vi "Get Target Info.vi"(8 "error in (no error)":errorcluster, 11 "FileOperation in":refnum<class "FileOperation.lvclass">) -> (0 "error out":errorcluster, 3 "FileOperation out":refnum<class "FileOperation.lvclass">)   [LabVIEW 2015, in "FileOperation.lvclass"]
uses:
  FileOperation.lvclass
  FileOperation.lvclass/FileOperation.ctl
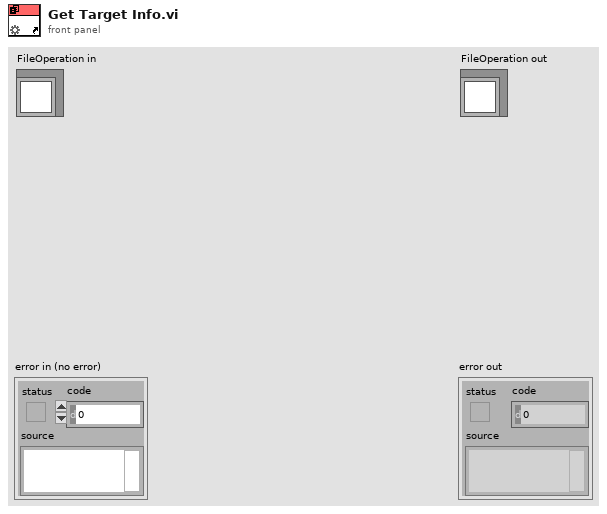
[diagram p1: front panel]
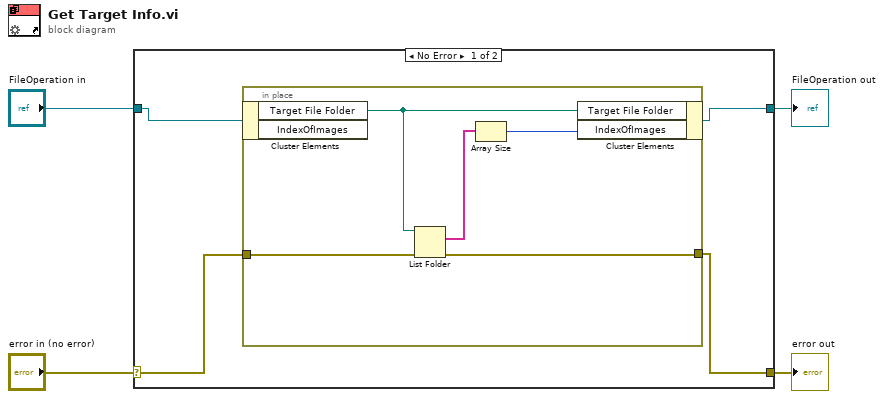
[diagram p0: block diagram]
diagram:
  n1 = case shown="No Error" "error in (no error)" {
    selector: "error in (no error)" -> [w8 w15]
    tunnel: [w6 w15] -> w3
    tunnel: [w5 w14] -> w1
    tunnel: "FileOperation in" -> [w7 w14]
    frame No Error {
      n2 = in-place {
        in-place-border: w8 -> [w13]
        in-place-border: [w10] -> w6
        n3 = in-place-cluster #1(w7) -> ("Target File Folder"=w12:path)  [unwired: 1 out]
        n4 = List Folder(path=w12, error in=w13) -> (filenames=w11:string[], error out=w10:errorcluster)  [unwired: 2 in, 2 out]
        n5 = Array Size(array=w11) -> (size(s)=w9:i32)
        n6 = in-place-cluster #1("Target File Folder"=w12, "IndexOfImages"=w9) -> (w5:refnum<class "FileOperation.lvclass">)
      }
    }
    frame Error {
    }
  }
  "error out" <- w3
  "FileOperation out" <- w1
